vi "Signal (SubVI).vi"(10 "Set? (T)":bool=TRUE, 11 "Occurrence in":refnum<k4>) -> ()   [LabVIEW 2017, in "SoC IP Library.lvlib"]
uses:
  SoC IP Library.lvlib
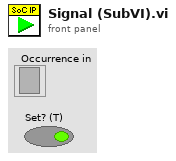
[diagram p1: front panel]
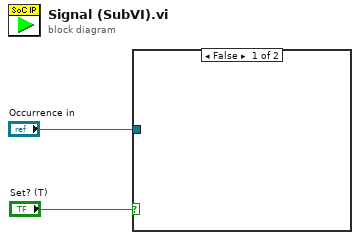
[diagram p0: block diagram]
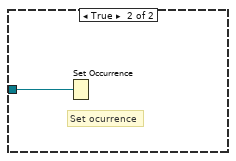
[diagram p2: hidden frame]
diagram:
  n1 = case shown="False" "Set? (T)" {
    tunnel: "Occurrence in" -> [_ w3]
    frame False {
    }
    frame True {
      # "Set ocurrence"
      n2 = Set Occurrence(w3) -> ()
    }
  }
